vi "NewtonsPSM_Sys_User_Para.vi"(0 "VISA session":refnum<visa-resource-name>, 1 "Phase Convention (0 to -360°)":u16(ring)=1 items=["-180° to 180°", "0 to -360°", "0 to 360°"], 11 "error in (no error)":errorcluster) -> (4 "dup VISA session":refnum<visa-resource-name>, 15 "error out":errorcluster)   [LabVIEW 2025, in "NewtonsPSM1735.lvlib"]
doc: "This VI set the General user parameters for the PPA2530"
uses:
  NewtonsPSM1735.lvlib
panel:
  in  "Control (V)":u16(ring) items=["V", "dBm"]
  in  "Step Message (On)":bool=TRUE
  in  "Autozero (Auto)":u16(ring) items=["Auto", "Manual"]
  in  "Keyboard Beep (On)":bool=TRUE
  in  "Graph Style (Lines)":u16(ring) items=["Lines", "Dots"]
  in  "Low Blanking (Off)":bool
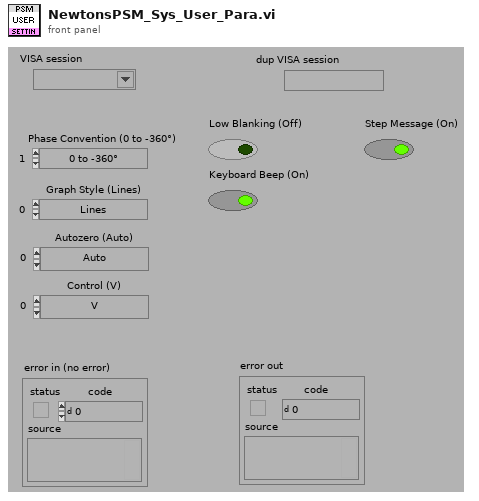
[diagram p1: front panel]
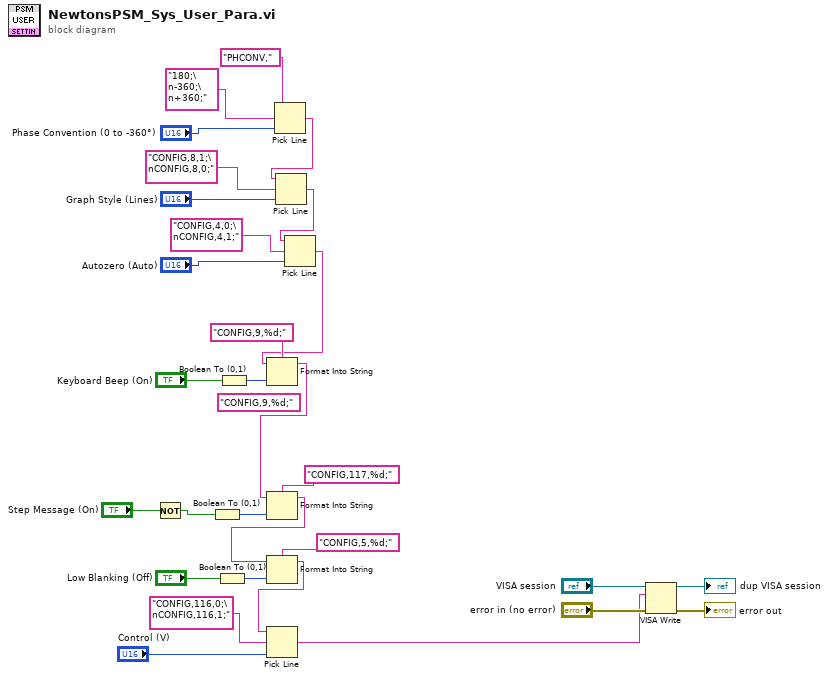
[diagram p0: block diagram]
diagram:
  (unwired) "CONFIG,9,%d;" ("format string")
  n1 = Not(x="Step Message (On)") -> (.not. x?=w3:bool)
  n2 = Boolean To (0,1)(Boolean=w3) -> (0, 1=w15:i16)
  n3 = Boolean To (0,1)(Boolean="Low Blanking (Off)") -> (0, 1=w14:i16)
  n4 = Boolean To (0,1)(Boolean="Keyboard Beep (On)") -> (0, 1=w17:i16)
  n5 = Pick Line(string ("")="PHCONV,", multi-line string="180;\n-360;\n+360;", line index="Phase Convention (0 to -360°)") -> (output string=w23:string)
  n6 = Pick Line(string ("")=w23, multi-line string="CONFIG,8,1;\nCONFIG,8,0;", line index="Graph Style (Lines)") -> (output string=w20:string)
  n7 = Pick Line(string ("")=w20, multi-line string="CONFIG,4,0;\nCONFIG,4,1;", line index="Autozero (Auto)") -> (output string=w7:string)
  n8 = Format Into String(format string="CONFIG,9,%d;", initial string=w7, w17) -> (resulting string=w6:string)  [unwired: 1 in, 1 out]
  n9 = Format Into String(format string="CONFIG,117,%d;", initial string=w6, w15) -> (resulting string=w9:string)  [unwired: 1 in, 1 out]
  n10 = Format Into String(format string="CONFIG,5,%d;", initial string=w9, w14) -> (resulting string=w2:string)  [unwired: 1 in, 1 out]
  n11 = Pick Line(string ("")=w2, multi-line string="CONFIG,116,0;\nCONFIG,116,1;" ("format string"), line index="Control (V)") -> (output string=w8:string)
  n12 = VISA Write(VISA resource name="VISA session", write buffer=w8, error in (no error)="error in (no error)") -> (VISA resource name out=→"dup VISA session":refnum<visa-resource-name>, error out=→"error out":errorcluster)  [unwired: 1 out]
